vi "ListTimePeroids.vi"(11 "UserEventTimer in":refnum<class "TimerEngine.lvclass">) -> (1 "TimePeroid":i64[](array[numeric]), 2 "Name":string[](array[string]), 3 "UserEventTimer out":refnum<class "TimerEngine.lvclass">)   [LabVIEW 2017, in "TimerEngine.lvlib" / "TimerEngine.lvclass"]
uses:
  TimerEngine.lvclass
  TimerEngine.lvclass/TimerEngine.ctl
  _TimerClass/Timer.lvclass/Timer.ctl
  _TimerClass/Timer.lvclass
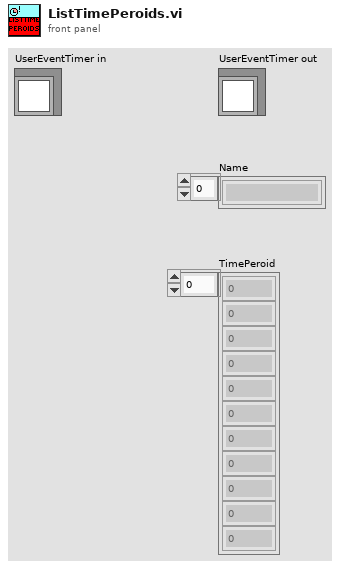
[diagram p1: front panel]
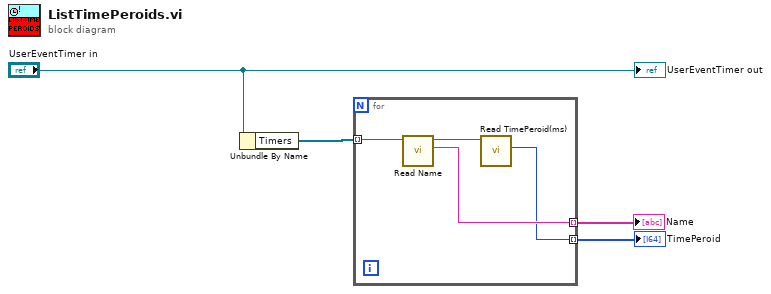
[diagram p0: block diagram]
diagram:
  n1 = Unbundle By Name("UserEventTimer in") -> ("Timers"=w3:refnum<class "Timer.lvclass">[])
  n2 = for {
    tunnel: w3 -> [w7] mode=indexing
    tunnel: [w6] -> w2 mode=indexing
    tunnel: [w5] -> w1 mode=indexing
    n3 = call "Read Name.vi"("Timer in"=w7) -> ("Name"=w6:string, "Timer out"=w8:refnum<class "Timer.lvclass">)  [unwired: 8 in, 1 out]
    n4 = call "Read TimePeroid(ms).vi"("Timer in"=w8) -> ("TimePeroid(ms)"=w5:i64)  [unwired: 8 in, 2 out]
  }
  "TimePeroid" <- w1
  "Name" <- w2
  "UserEventTimer out" <- "UserEventTimer in"
